vi "Main GUI.vi"() -> ()   [LabVIEW 2018]
uses:
  Button Class/Button Handler State.ctl
  Button Class/TCP Multiple Connections Data.ctl
  Button Class/TCP Multiple Connections State.ctl
  Button Class/Button.lvclass
panel:
  in  "Stop":bool
  out "T3A1/A2":bool
  out "T3A13/A14":bool
  out "T3A11/A12":bool
  out "T3A9/A10":bool
  out "T3A8":bool
  out "T3A7":bool
  out "T3A5/A6":bool
  out "T3A3/A4":bool
  out "192.168.1.163":bool
  out "192.168.1.162":bool
  out "192.168.1.161":bool
  out "192.168.3.160":bool
  out "192.168.3.159":bool
  out "192.168.3.158":bool
  out "192.168.3.157":bool
  out "192.168.3.156":bool
  out "192.168.3.155":bool
  out "192.168.3.154":bool
  out "192.168.3.153":bool
  out "192.168.3.152":bool
  out "192.168.3.151":bool
  out "192.168.3.150":bool
  out "192.168.3.149":bool
  out "192.168.3.148":bool
  out "192.168.3.147":bool
  out "192.168.3.146":bool
  out "192.168.3.145":bool
  out "192.168.3.144":bool
  out "192.168.3.143":bool
  out "192.168.3.142":bool
  out "192.168.3.141":bool
  out "192.168.3.140":bool
  out "192.168.3.139":bool
  out "192.168.3.138":bool
  out "192.168.3.137":bool
  out "192.168.3.136":bool
  out "192.168.3.135":bool
  out "192.168.3.134":bool
  out "192.168.3.133":bool
  out "192.168.3.132":bool
  out "192.168.3.131":bool
  out "192.168.3.130":bool
  out "192.168.3.129":bool
  out "192.168.3.128":bool
  out "192.168.3.127":bool
  out "192.168.3.126":bool
  out "192.168.3.125":bool
  out "192.168.3.124":bool
  out "192.168.3.123":bool
  out "192.168.3.122":bool
  out "192.168.3.121":bool
  out "192.168.3.120":bool
  out "192.168.3.119":bool
  out "192.168.3.118":bool
  out "192.168.3.117":bool
  out "192.168.3.116":bool
  out "192.168.3.115":bool
  out "192.168.3.114":bool
  out "192.168.3.113":bool
  out "192.168.3.112":bool
  out "192.168.3.111":bool
  out "192.168.3.110":bool
  out "192.168.3.109":bool
  out "error out":errorcluster
  in  "error in (no error)":errorcluster
  # "G1/G2"
  # "F1/F2"
  # "E1/E2"
  # "D1/D2"
  # "C1/C2"
  # "B1/B2"
  # "I1/I2"
  # "A1/A2"
  # "H1"
  # "G3/G4"
  # "F3/F4"
  # "E3/E4"
  # "D3/D4"
  # "C3/C4"
  # "B3/B4"
  # "A3/A4"
  # "I3/I4"
  # "H3"
  # "D5/D6"
  # "A5/A6"
  # "G5/G6"
  # "F5/F6"
  # "E5/E6"
  # "C5/C6"
  # "B5/B6"
  # "I5"
  # "B5/B6"
  # "D7"
  # "A7"
  # "G7"
  # "E7"
  # "C7"
  # "B7"
  # "F7"
  # "G8"
  # "F8"
  # "E8"
  # "D8"
  # "C8"
  # "B8"
  # "A8"
  # "G9/G10"
  # "F9/F10"
  # "E9/E10"
  # "D9/D10"
  # "C9/C10"
  # "B9/B10"
  # "A9/A10"
  # "H4"
  # "A11/A12"
  # "G11/G12"
  # "F11/F12"
  # "E11/E12"
  # "D11/D12"
  # "C11/C12"
  # "B11/B12"
  # "H6"
  # "G13/G14"
  # "F13/F14"
  # "E13/E14"
  # "D13/D14"
  # "C13/C14"
  # "B13/B14"
  # "A13/A14"
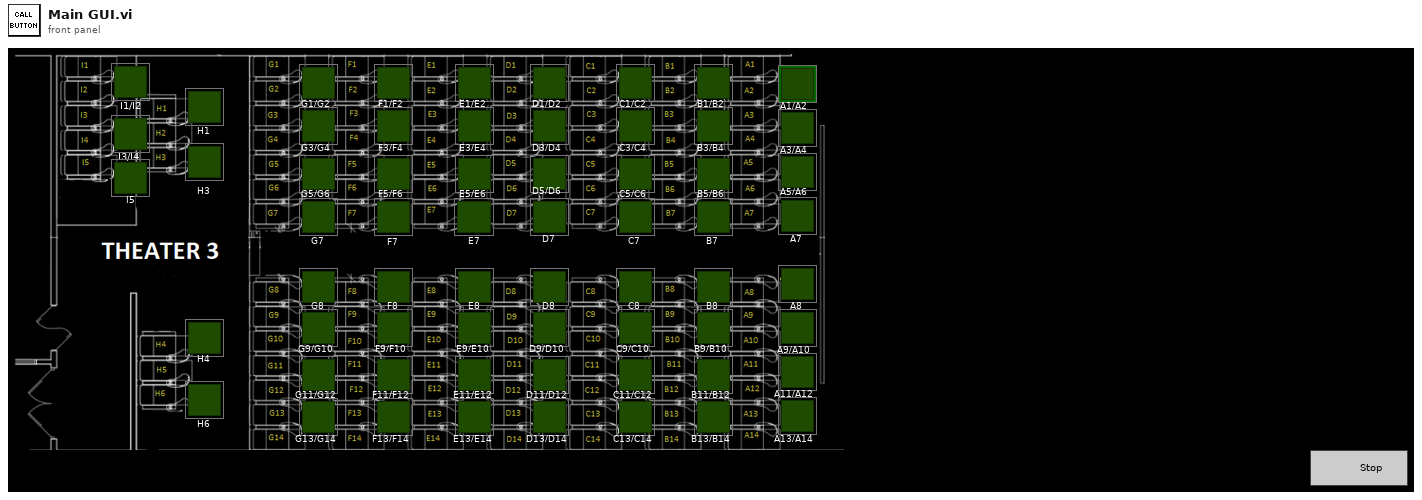
[diagram p1: front panel]
types:
  T1 = typedef "TCP Multiple Connections State.ctl" = enum16{"Initialize", "Status Check", "Read Data", "Stop"}
  T2 = typedef "TCP Multiple Connections Data.ctl" = cluster{"Clients":refnum<k5>[], "Listener":refnum<k5>}
  T3 = typedef "Button Handler State.ctl" = enum16{"Initialize", "Check Active", "Update Colors", "Message Check"}
  T4 = enum16{"Standard", "Buffered", "CRLF", "Immediate"}
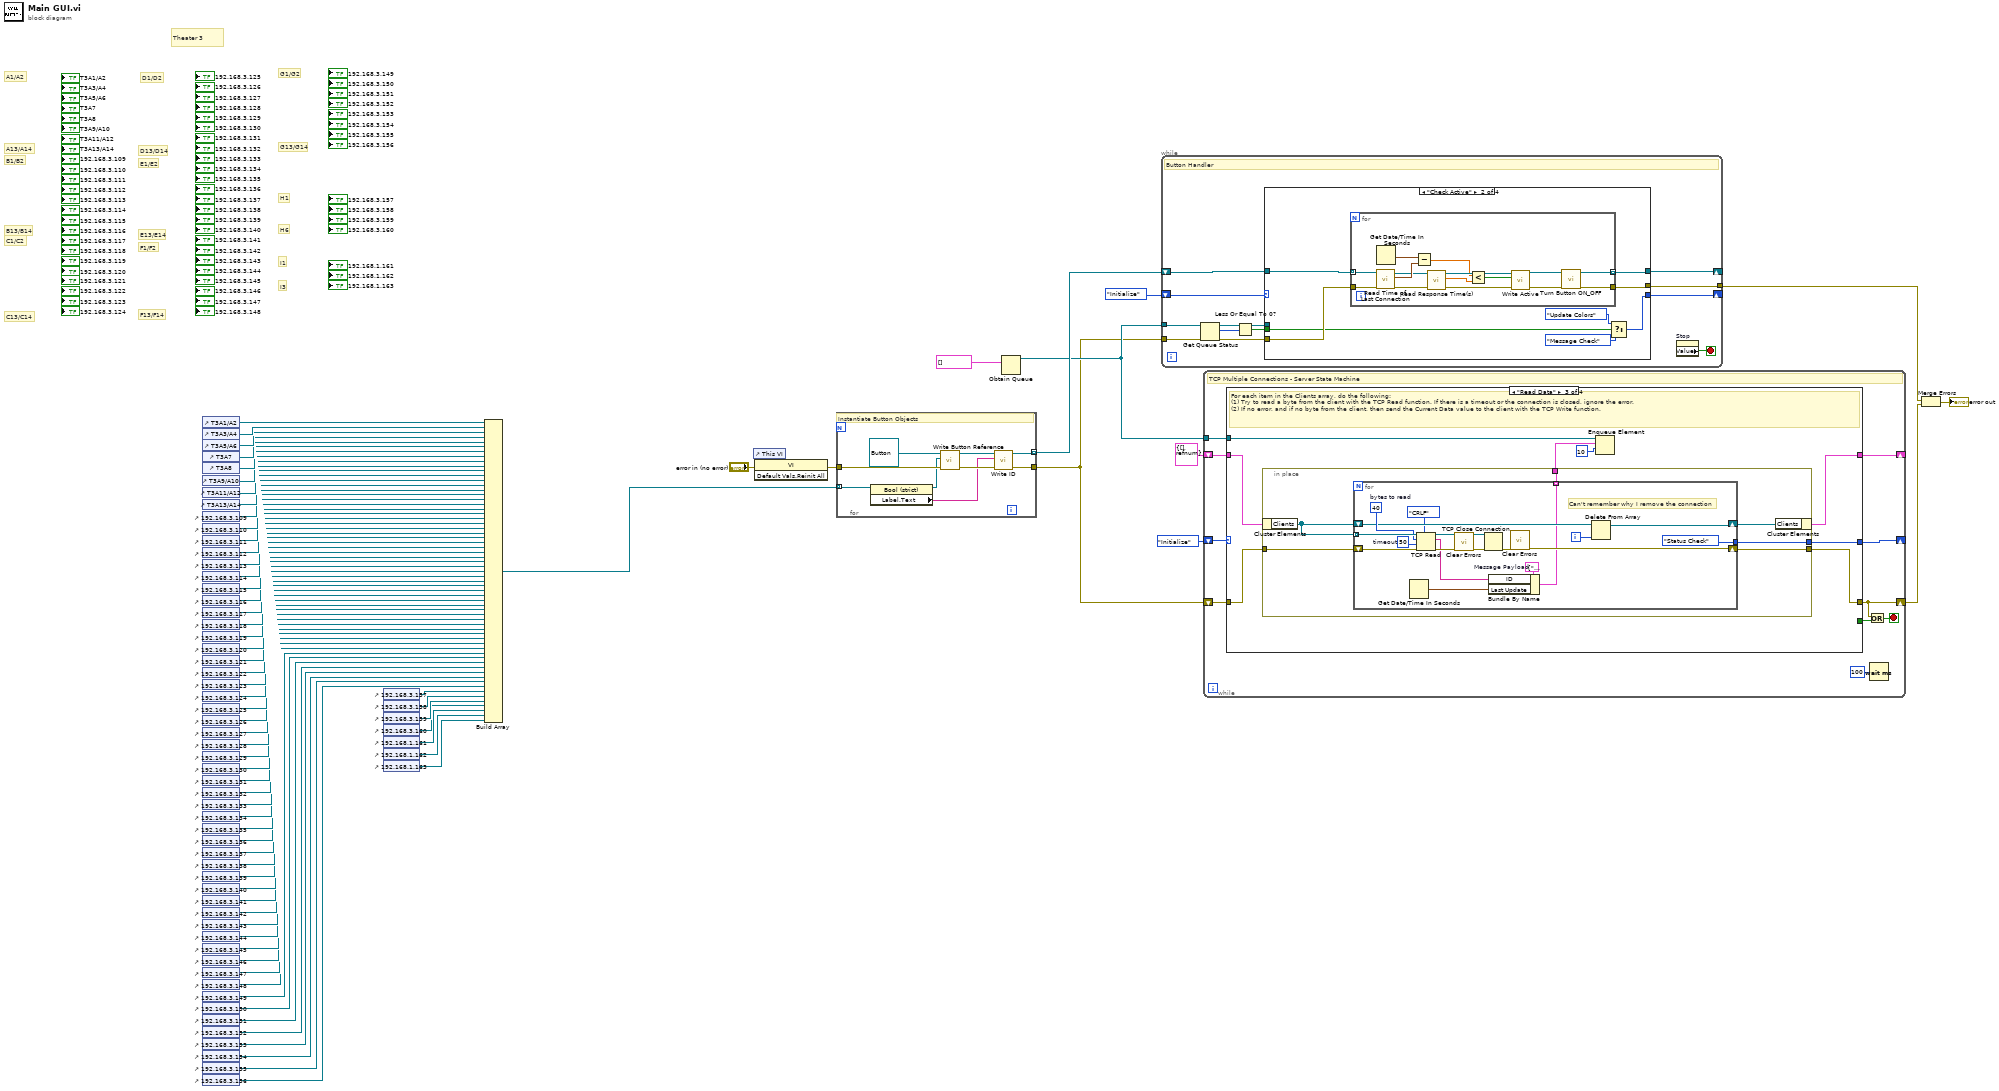
[diagram p0: block diagram]
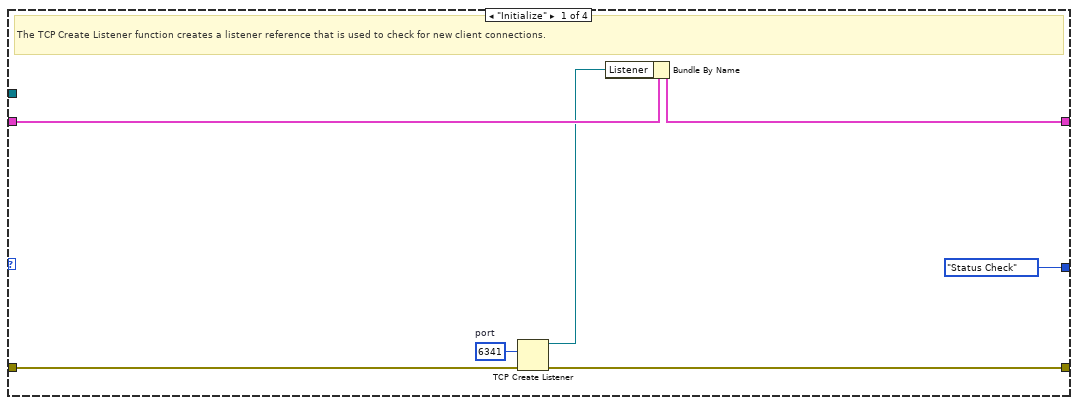
[diagram p2: hidden frame]
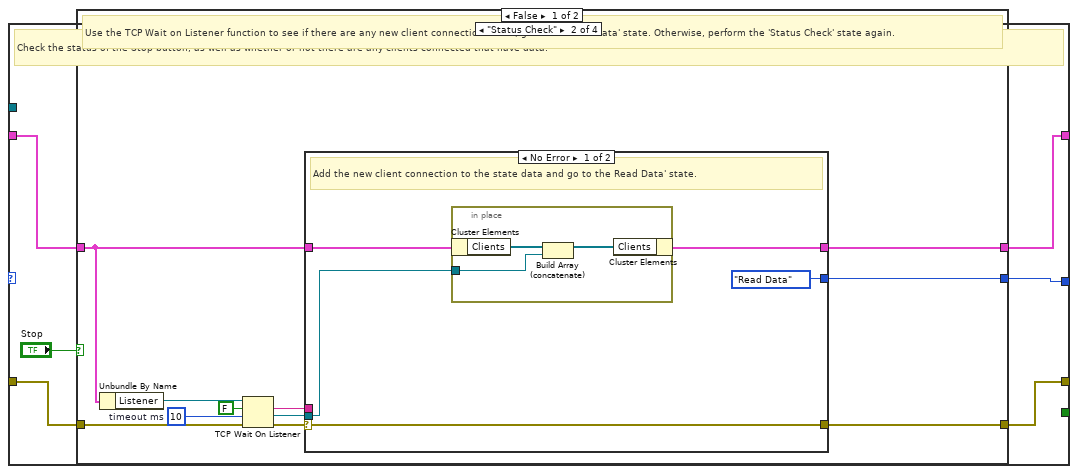
[diagram p3: hidden frame]
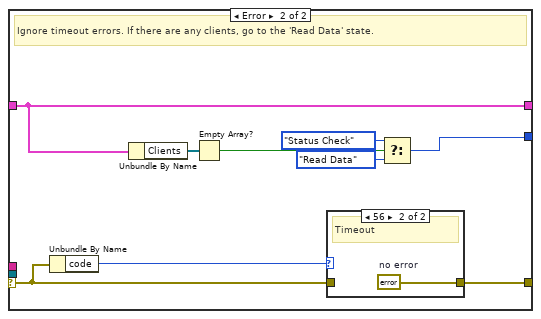
[diagram p4: hidden frame]
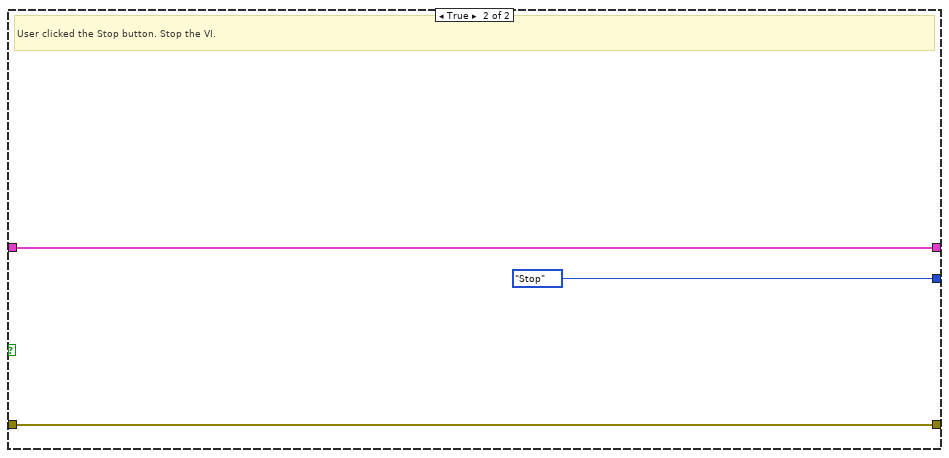
[diagram p6: hidden frame]
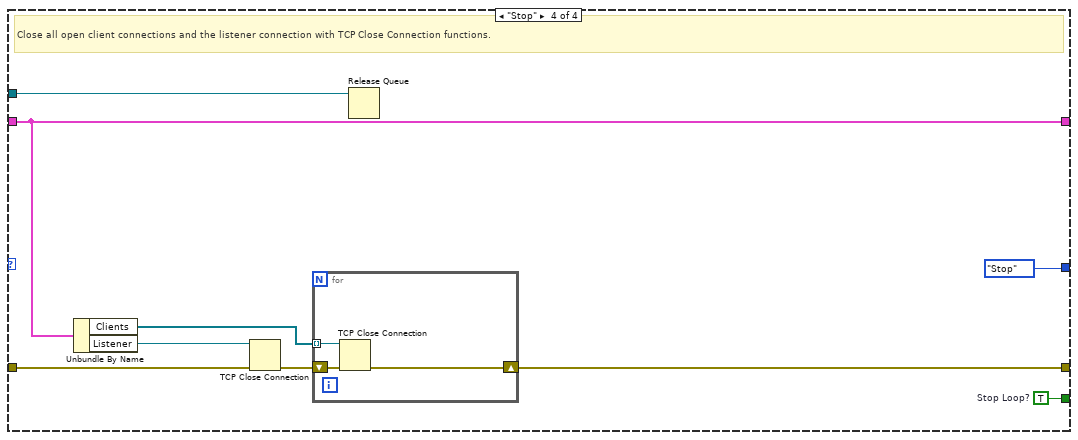
[diagram p7: hidden frame]
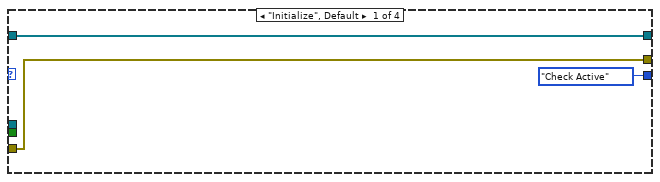
[diagram p8: hidden frame]
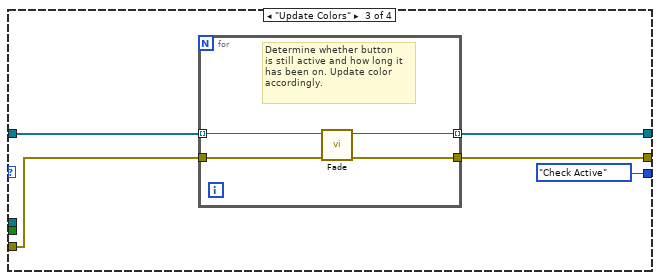
[diagram p9: hidden frame]
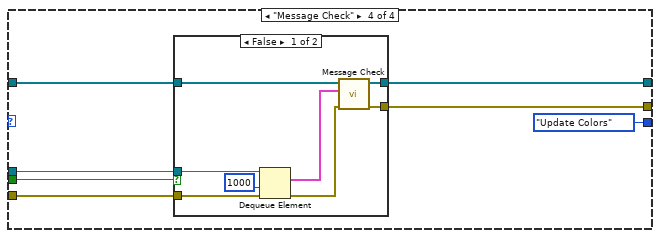
[diagram p10: hidden frame]
diagram:
  # "G13/G14"
  # "H6"
  # "I3"
  # "I1"
  # "H1"
  # "G1/G2"
  # "F13/F14"
  # "F1/F2"
  # "E13/E14"
  # "E1/E2"
  # "D1/D2"
  # "D13/D14"
  # "C13/C14"
  # "C1/C2"
  # "B13/B14"
  # "B1/B2"
  # "A13/A14"
  # "A1/A2"
  # "Theater 3"
  n1 = control-ref of="T3A1/A2"() -> (w5:refnum<vi>)
  n2 = control-ref of="T3A3/A4"() -> (w77:refnum<vi>)
  n3 = control-ref of="T3A5/A6"() -> (w76:refnum<vi>)
  n4 = control-ref of="T3A7"() -> (w75:refnum<vi>)
  n5 = control-ref of="T3A8"() -> (w74:refnum<vi>)
  n6 = control-ref of="T3A9/A10"() -> (w69:refnum<vi>)
  n7 = control-ref of="T3A11/A12"() -> (w68:refnum<vi>)
  n8 = control-ref of="T3A13/A14"() -> (w67:refnum<vi>)
  n9 = control-ref of="192.168.3.109"() -> (w66:refnum<vi>)
  n10 = control-ref of="192.168.3.110"() -> (w65:refnum<vi>)
  n11 = control-ref of="192.168.3.111"() -> (w64:refnum<vi>)
  n12 = control-ref of="192.168.3.112"() -> (w63:refnum<vi>)
  n13 = control-ref of="192.168.3.113"() -> (w62:refnum<vi>)
  n14 = control-ref of="192.168.3.114"() -> (w61:refnum<vi>)
  n15 = control-ref of="192.168.3.115"() -> (w60:refnum<vi>)
  n16 = control-ref of="192.168.3.116"() -> (w59:refnum<vi>)
  n17 = control-ref of="192.168.3.117"() -> (w58:refnum<vi>)
  n18 = control-ref of="192.168.3.118"() -> (w57:refnum<vi>)
  n19 = control-ref of="192.168.3.119"() -> (w56:refnum<vi>)
  n20 = control-ref of="192.168.3.120"() -> (w55:refnum<vi>)
  n21 = control-ref of="192.168.3.121"() -> (w54:refnum<vi>)
  n22 = control-ref of="192.168.3.122"() -> (w53:refnum<vi>)
  n23 = control-ref of="192.168.3.123"() -> (w52:refnum<vi>)
  n24 = control-ref of="192.168.3.124"() -> (w51:refnum<vi>)
  n25 = control-ref of="192.168.3.125"() -> (w50:refnum<vi>)
  n26 = control-ref of="192.168.3.126"() -> (w49:refnum<vi>)
  n27 = control-ref of="192.168.3.127"() -> (w48:refnum<vi>)
  n28 = control-ref of="192.168.3.128"() -> (w47:refnum<vi>)
  n29 = control-ref of="192.168.3.129"() -> (w46:refnum<vi>)
  n30 = control-ref of="192.168.3.130"() -> (w45:refnum<vi>)
  n31 = control-ref of="192.168.3.131"() -> (w44:refnum<vi>)
  n32 = control-ref of="192.168.3.132"() -> (w43:refnum<vi>)
  n33 = control-ref of="192.168.3.133"() -> (w42:refnum<vi>)
  n34 = control-ref of="192.168.3.134"() -> (w41:refnum<vi>)
  n35 = control-ref of="192.168.3.135"() -> (w40:refnum<vi>)
  n36 = control-ref of="192.168.3.136"() -> (w39:refnum<vi>)
  n37 = control-ref of="192.168.3.137"() -> (w38:refnum<vi>)
  n38 = control-ref of="192.168.3.138"() -> (w37:refnum<vi>)
  n39 = control-ref of="192.168.3.139"() -> (w36:refnum<vi>)
  n40 = control-ref of="192.168.3.140"() -> (w35:refnum<vi>)
  n41 = control-ref of="192.168.3.141"() -> (w34:refnum<vi>)
  n42 = control-ref of="192.168.3.142"() -> (w33:refnum<vi>)
  n43 = control-ref of="192.168.3.143"() -> (w32:refnum<vi>)
  n44 = control-ref of="192.168.3.144"() -> (w31:refnum<vi>)
  n45 = control-ref of="192.168.3.145"() -> (w30:refnum<vi>)
  n46 = control-ref of="192.168.3.146"() -> (w29:refnum<vi>)
  n47 = control-ref of="192.168.3.147"() -> (w28:refnum<vi>)
  n48 = control-ref of="192.168.3.148"() -> (w27:refnum<vi>)
  n49 = control-ref of="192.168.3.149"() -> (w26:refnum<vi>)
  n50 = control-ref of="192.168.3.150"() -> (w25:refnum<vi>)
  n51 = control-ref of="192.168.3.151"() -> (w24:refnum<vi>)
  n52 = control-ref of="192.168.3.152"() -> (w23:refnum<vi>)
  n53 = control-ref of="192.168.3.153"() -> (w22:refnum<vi>)
  n54 = control-ref of="192.168.3.154"() -> (w21:refnum<vi>)
  n55 = control-ref of="192.168.3.155"() -> (w20:refnum<vi>)
  n56 = control-ref of="192.168.3.156"() -> (w19:refnum<vi>)
  n57 = control-ref of="192.168.3.157"() -> (w18:refnum<vi>)
  n58 = control-ref of="192.168.3.158"() -> (w17:refnum<vi>)
  n59 = control-ref of="192.168.3.159"() -> (w16:refnum<vi>)
  n60 = control-ref of="192.168.3.160"() -> (w15:refnum<vi>)
  n61 = control-ref of="192.168.1.161"() -> (w14:refnum<vi>)
  n62 = control-ref of="192.168.1.162"() -> (w13:refnum<vi>)
  n63 = control-ref of="192.168.1.163"() -> (w12:refnum<vi>)
  n64 = Build Array(w5, w77, w76, w75, w74, w69, w68, w67, w66, w65, w64, w63, w62, w61, w60, w59, w58, w57, w56, w55, w54, w53, w52, w51, w50, w49, w48, w47, w46, w45, w44, w43, w42, w41, w40, w39, w38, w37, w36, w35, w34, w33, w32, w31, w30, w29, w28, w27, w26, w25, w24, w23, w22, w21, w20, w19, w18, w17, w16, w15, w14, w13, w12) -> (w73:refnum<vi>[])
  n65 = control-ref of="This VI"() -> (w72:refnum<vi>)
  n66 = invoke class="VI" method="Default Vals.Reinit All"(reference=w72, error in="error in (no error)") -> (error out=w70:errorcluster)  [unwired: 1 in, 2 out]
  n67 = for {
    tunnel: w73 -> [w78] mode=indexing
    tunnel: [w81] -> w4 mode=indexing
    tunnel: w70 -> [w85]
    tunnel: [w80] -> w1
    # "Instantiate Button Objects"
    n68 = property class="Bool (strict)"(reference=w78) -> (reference out=w79:refnum<vi>, "Label.Text"=w82:string)  [unwired: 1 in, 1 out]
    n69 = call-dynamic "Write Button Reference.vi"("error in (no error)"=w85, "Button Reference"=w79, "Button in"=refnum<class "Button.lvclass"> refnum ("Button.lvclass")) -> ("error out"=w83:errorcluster, "Button out"=w84:refnum<class "Button.lvclass">)  [unwired: 7 in]
    n70 = call-dynamic "Write ID.vi"("error in (no error)"=w83, "ID"=w82, "Button in"=w84) -> ("error out"=w80:errorcluster, "Button out"=w81:refnum<class "Button.lvclass">)  [unwired: 7 in]
  }
  n71 = Obtain Queue(element data type=cluster{"ID":string, "current time":timestamp}[] [] ("element")) -> (queue out=w2:refnum<queue>)  [unwired: 4 in, 2 out]
  n72 = while {
    shift-right: [w97] -> _
    shift-left: Button_Handler_State."Initialize" -> [w98]
    tunnel: [w96] -> w10
    shift-right: [w93] -> _
    shift-left: w4 -> [w94]
    tunnel: w2 -> [w92]
    tunnel: w1 -> [w89]
    stop <- w95 stop-if-true
    # "Button Handler"
    n73 = Get Queue Status(queue=w92, error in (no error)=w89) -> (queue out=w91:refnum<queue>, error out=w88:errorcluster, # elements in queue=w87:i32)  [unwired: 1 in, 5 out]
    n74 = Less Or Equal To 0?(x=w87) -> (x <= 0?=w90:bool)
    n75 = case shown="\"Check Active\"" w98 {
      tunnel: w94 -> [w100 w109 w129 w140]
      tunnel: [Button_Handler_State."Check Active" w105 Button_Handler_State."Check Active" Button_Handler_State."Update Colors"] -> w97
      tunnel: [w99 w108 w128 w139] -> w96
      tunnel: [w100 w104 w126 w137] -> w93
      tunnel: w91 -> [_ _ _ w136]
      tunnel: w90 -> [_ w102 _ w135]
      tunnel: w88 -> [w99 w103 w125 w134]
      frame "Initialize", Default {
      }
      frame "Check Active" {
        n76 = for {
          tunnel: w109 -> [w124] mode=indexing
          tunnel: [w113] -> w108
          tunnel: [w111] -> w104 mode=indexing
          tunnel: w103 -> [w110]
          n77 = call-dynamic "Read Time of Last Connection.vi"("error in (no error)"=w110, "Button in"=w124) -> ("error out"=w117:errorcluster, "Time of Last Connection"=w122:timestamp, "Button out"=w120:refnum<class "Button.lvclass">)  [unwired: 7 in]
          n78 = Get Date/Time In Seconds() -> (seconds since 1Jan1904=w123:timestamp)
          n79 = Subtract(x=w123, y=w122) -> (x-y=w115:dbl)
          n80 = call-dynamic "Read Response Time(s).vi"("error in (no error)"=w117, "Button in"=w120) -> ("error out"=w116:errorcluster, "Response Time(s)"=w118:dbl, "Button out"=w119:refnum<class "Button.lvclass">)  [unwired: 7 in]
          n81 = Less?(x=w115, y=w118) -> (x < y?=w121:bool)
          n82 = call-dynamic "Write Active.vi"("error in (no error)"=w116, "Active"=w121, "Button in"=w119) -> ("error out"=w112:errorcluster, "Button out"=w114:refnum<class "Button.lvclass">)  [unwired: 7 in]
          n83 = call "Turn Button ON_OFF.vi"("error in (no error)"=w112, "Button in"=w114) -> ("error out"=w113:errorcluster, "Button out"=w111:refnum<class "Button.lvclass">)  [unwired: 8 in]
        }
        n84 = Select(t=Button_Handler_State."Update Colors", s=w102, f=Button_Handler_State."Message Check") -> (s? t:f=w105:T3)
      }
      frame "Update Colors" {
        n85 = for {
          tunnel: w129 -> [w132] mode=indexing
          tunnel: [w133] -> w128
          tunnel: [w131] -> w126 mode=indexing
          tunnel: w125 -> [w130]
          # "Determine whether button\nis still active and how long it\nhas been on. Update color \naccordingly."
          n86 = call "Fade.vi"("error in (no error)"=w130, "Button in"=w132) -> ("error out"=w133:errorcluster, "Button out"=w131:refnum<class "Button.lvclass">)  [unwired: 8 in]
        }
      }
      frame "Message Check" {
        n87 = case shown="False" w135 {
          tunnel: w140 -> [w148 w150]
          tunnel: [w147 w149] -> w139
          tunnel: [w146 w150] -> w137
          tunnel: w136 -> [w145 _]
          tunnel: w134 -> [w142 w149]
          frame False {
            n88 = Dequeue Element(queue=w145, timeout in ms (-1)=1000, error in (no error)=w142) -> (element=w143:cluster{"ID":string, "current time":timestamp}[], error out=w141:errorcluster)  [unwired: 2 out]
            n89 = call "Message Check.vi"("error in (no error)"=w141, "element"=w143, "Array in"=w148) -> ("error out"=w147:errorcluster, "Array"=w146:refnum<class "Button.lvclass">[])  [unwired: 7 in]
          }
          frame True {
          }
        }
      }
    }
    n90 = property on="Stop" class="Bool (strict)"() -> ("Value"=w95:bool)  [unwired: 2 in, 2 out]
  }
  n91 = while {
    shift-right: [w153] -> _
    shift-left: TCP_Multiple_Connections_State."Initialize" ("States") -> [w160]
    shift-right: [w158] -> _
    shift-left: T2 {"Clients"=[], "Listener"=refnum} ("Data") -> [w159]
    shift-right: [w154] -> w6
    shift-left: w1 -> [w157]
    tunnel: w2 -> [w152]
    stop <- w155 stop-if-true
    # "TCP Multiple Connections - Server State Machine"
    n92 = case shown="\"Read Data\"" w160 {
      tunnel: [TCP_Multiple_Connections_State."Status Check" ("States") w173 w210 TCP_Multiple_Connections_State."Stop" ("(Value Not Used)")] -> w153
      tunnel: [_ _ _ w247] -> w156
      tunnel: w159 -> [w165 w169 w212 w246]
      tunnel: [w164 w168 w211 w246] -> w158
      tunnel: w157 -> [w167 w172 w214 w245]
      tunnel: [w166 w171 w213 w243] -> w154
      tunnel: w152 -> [_ _ w209 w239]
      frame "Initialize" {
        w162 = u16 6341  # port
        # "The TCP Create Listener function creates a listener reference that is used to check for new client connections."
        n93 = TCP Create Listener(8:w167, 10:w162) -> (0:w166:errorcluster, 3:w163:refnum<k5>)  [unwired: 4 out]
        n94 = Bundle By Name(cluster=w165, "Listener"=w163) -> (w164:T2)
      }
      frame "Status Check" {
        # "Check the status of the Stop button, as well as whether or not there are any clients connected that have data."
        n95 = case shown="False" "Stop" {
          tunnel: [w184 TCP_Multiple_Connections_State."Stop" ("States")] -> w173
          tunnel: w172 -> [w183 w206]
          tunnel: [w176 w206] -> w171
          tunnel: w169 -> [w179 w205]
          tunnel: [w178 w205] -> w168
          frame False {
            w182 = 10  # timeout ms
            # "Use the TCP Wait on Listener function to see if there are any new client connections. If so, go to the Read Data' state. Otherwise, perform the 'Status Check' state again."
            n96 = Unbundle By Name(w179) -> ("Listener"=w177:refnum<k5>)
            n97 = TCP Wait On Listener(8:w183, 9:w182, 10:FALSE ("resolve remote address (T)"), 11:w177) -> (0:w181:errorcluster, 2:w175:string, 4:w180:refnum<k5>)  [unwired: 2 out]
            n98 = case shown="No Error" w181 {
              selector: w181 -> [w187 w201]
              tunnel: [TCP_Multiple_Connections_State."Read Data" ("Initial State") w195] -> w184
              tunnel: w180 -> [w188 _]
              tunnel: w179 -> [w189 w198]
              tunnel: [w186 w198] -> w178
              tunnel: [w187 w199] -> w176
              tunnel: w175 -> [_ _]
              frame No Error {
                # "Add the new client connection to the state data and go to the Read Data' state."
                n99 = in-place {
                  in-place-border: w188 -> [w190]
                  n100 = in-place-cluster #1(w189) -> ("Clients"=w192:refnum<k5>[])
                  n101 = Build Array (concatenate)(w192, w190) -> (w191:refnum<k5>[])
                  n102 = in-place-cluster #1("Clients"=w191) -> (w186:T2)
                }
              }
              frame Error {
                # "Ignore timeout errors. If there are any clients, go to the 'Read Data' state."
                n103 = Unbundle By Name(w201) -> ("code"=w200:i32)
                n104 = Unbundle By Name(w198) -> ("Clients"=w197:refnum<k5>[])
                n105 = Empty Array?(array=w197) -> (empty?=w196:bool)
                n106 = case shown="56" w200 {
                  tunnel: w201 -> [w202 _]
                  tunnel: [w202 w203] -> w199
                  frame Default {
                  }
                  frame 56 {
                    w203 = errorcluster {"status"=FALSE, "code"=0, "source"=""}  # no error
                    # "Timeout"
                  }
                }
                n107 = Select(t=TCP_Multiple_Connections_State."Status Check" ("States"), s=w196, f=TCP_Multiple_Connections_State."Read Data" ("Initial State")) -> (s? t:f=w195:T1)
              }
            }
          }
          frame True {
            # "User clicked the Stop button. Stop the VI."
          }
        }
      }
      frame "Read Data" {
        # "For each item in the Clients array, do the following:\n(1) Try to read a byte from the client with the TCP Read function. If there is a timeout or the connection is closed, ignore the error. \n(2) If no error, and if no byte from the client, then send the Current Data value to the client with the TCP Write function."
        n108 = in-place {
          in-place-border: w214 -> [w220]
          in-place-border: [w219] -> w213
          in-place-border: [w218] -> w210
          in-place-border: [w215] -> w207
          n109 = in-place-cluster #2(w212) -> ("Clients"=w216:refnum<k5>[])
          n110 = for {
            tunnel: w216 -> [w238] mode=indexing
            shift-right: [w234] -> w219
            shift-left: w220 -> [w236]
            tunnel: [TCP_Multiple_Connections_State."Status Check" ("States")] -> w218
            shift-right: [w230] -> w217
            shift-left: w216 -> [w229]
            tunnel: [w221] -> w215 mode=indexing
            i -> [w225]
            w222 = cluster{"ID":string, "Last Update":timestamp} {"ID"="", "Last Update"=timestamp(0 s since 1904-01-01)}  # Message Payload
            w237 = 50  # timeout
            w233 = 40  # bytes to read
            # "Can't remember why I remove the connection"
            n111 = Get Date/Time In Seconds() -> (seconds since 1Jan1904=w223:timestamp)
            n112 = TCP Read(connection ID=w238, bytes to read=w233, error in (no error)=w236, 7:T4."CRLF" ("mode (standard)"), 9:w237) -> (connection ID out=w235:refnum<k5>, data out=w224:string, error out=w232:errorcluster)
            n113 = call <vilib>:"Clear Errors.vi"("error in (no error)"=w232) -> ("error out"=w228:errorcluster)  [unwired: 5 in, 1 out]
            n114 = TCP Close Connection(connection ID=w235, error in (no error)=w228) -> (error out=w227:errorcluster)  [unwired: 1 in, 1 out]
            n115 = Bundle By Name(cluster=w222, "ID"=w224, "Last Update"=w223) -> (w221:cluster{"ID":string, "Last Update":timestamp})
            n116 = call <vilib>:"Clear Errors.vi"("error in (no error)"=w227) -> ("error out"=w234:errorcluster)  [unwired: 5 in, 1 out]
            n117 = Delete From Array(array=w229, index=w225) -> (array with subset deleted=w230:refnum<k5>[])  [unwired: 1 in, 1 out]
          }
          n118 = in-place-cluster #2("Clients"=w217) -> (w211:T2)
        }
        n119 = Enqueue Element(queue=w209, element=w207, timeout in ms (-1)=10) -> ()  [unwired: 1 in, 3 out]
      }
      frame "Stop" {
        w247 = TRUE  # Stop Loop?
        # "Close all open client connections and the listener connection with TCP Close Connection functions."
        n120 = Unbundle By Name(w246) -> ("Clients"=w244:refnum<k5>[], "Listener"=w241:refnum<k5>)
        n121 = TCP Close Connection(connection ID=w241, error in (no error)=w245) -> (error out=w242:errorcluster)  [unwired: 1 in, 1 out]
        n122 = for {
          shift-right: [w249] -> w243
          shift-left: w242 -> [w250]
          tunnel: w244 -> [w248] mode=indexing
          n123 = TCP Close Connection(connection ID=w248, error in (no error)=w250) -> (error out=w249:errorcluster)  [unwired: 1 in, 1 out]
        }
        n124 = Release Queue(queue=w239) -> ()  [unwired: 2 in, 3 out]
      }
    }
    n125 = Or(x=w154, y=w156) -> (x .or. y?=w155:bool)
    n126 = Wait (ms)(milliseconds to wait=u32 100) -> ()  [unwired: 1 out]
  }
  n127 = Merge Errors(w10, w6) -> (→"error out":errorcluster)
